vi "XY Graph Add Multiplots with Names v2.vi"(0 "XYGraph in":T3, 1 "Array of Scales (Default)":cluster{"X Scale":u32, "Y Scale":u32}[](array[cluster]), 2 "Plots Interpolation (Previous Plot's Style)":T2[](array[typedef]), 3 "Keep Existing Plots (T)":bool=TRUE, 5 "Array of Plots":cluster{"X Array":dbl[], "Y Array":dbl[]}[](array[cluster]), 7 "Plots Metadata":variant[](array[variant]), 9 "Array of Plot Names (\"Plot\")":string[](array[string]), 11 "error in (no error)":errorcluster, 12 "Make Visible (T)":bool=TRUE, 13 "Plot Colors (Default)":u32[](array[colorbox]), 14 "Point Style (Dot)":T1=enum."Dot") -> (4 "XY Graph Caption (or Label)":string, 6 "Total Number of Plots":i32, 8 "Number of Plots Added":i32, 10 "Added Plot Names":string[](array[string]), 15 "error out":errorcluster)   [LabVIEW 2021, in "XY Graph Add-Ons.lvlib"]
uses:
  XY Graph Add-Ons.lvlib
  XY Graph Refnum.ctl
  LabVIEW Plot Interpolation.ctl
  Plot Point Style.ctl
  XY Graph Get Plots Metadata.vi
  XY Graph Set Plots Metadata.vi
  Strings/Strings.lvlib
  Graphs.lvlib
  Error/Error.lvlib
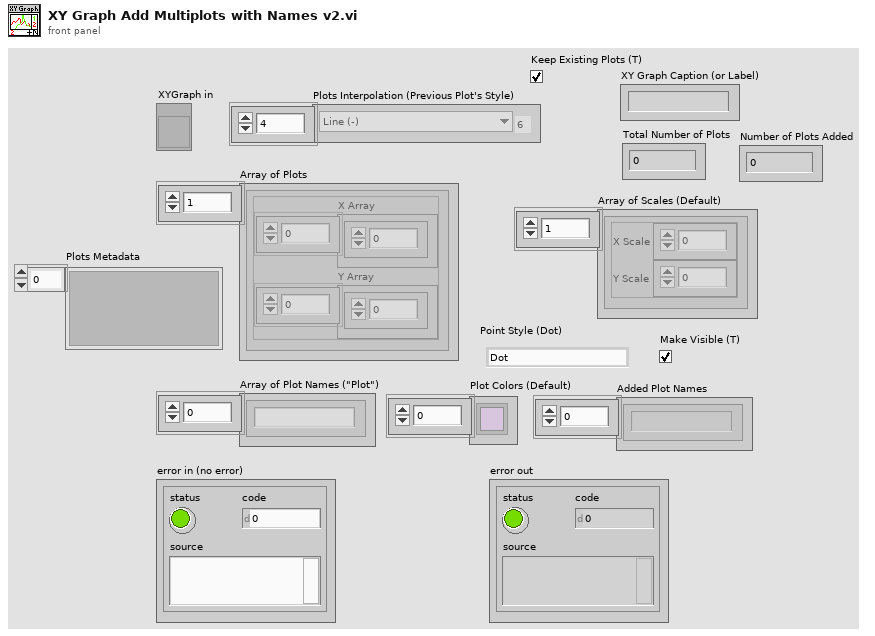
[diagram p1: front panel]
types:
  T1 = typedef "Graphs.lvlib/Plot Point Style.ctl" = enum16{"not defined", "None", "Empty Circle", "Filled Circle", "Thick Circle", "Dotted Circle", "Empty Square", "Filled Square", "Thick Square", "Dotted Square", "Small Filled Square", "Dot", "Cross", "Tiny Cross", "Large X", "Small x", "Diamond", "Small Empty Square"}
  T2 = typedef "Graphs.lvlib/LabVIEW Plot Interpolation.ctl" = enum16{"Point (.)", "Stepwise Right (--.)", "Line + Point (\\. /)", "Stepwise Left (.--)", "Stepwise Centered (-.-)", "Stepwise Vertical (|.|)", "Line (-)", "Use Previous Plot's Style"}
  T3 = typedef "XY Graph Add-Ons.lvlib/XY Graph Refnum.ctl" = refnum<vi>
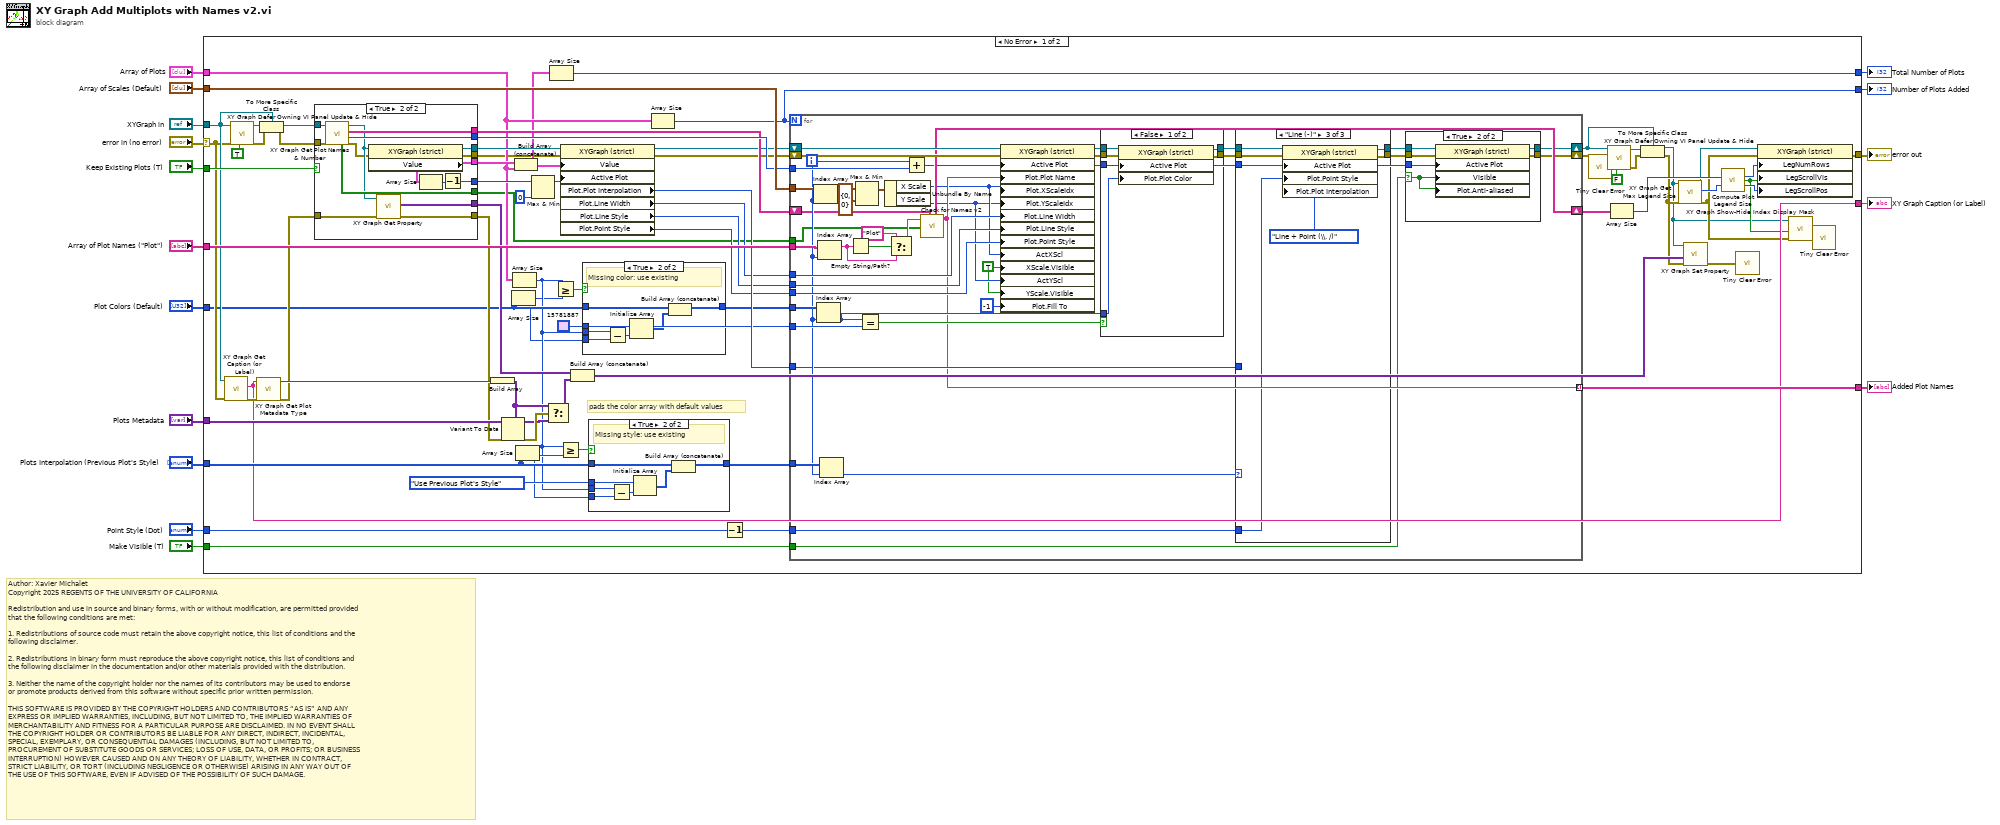
[diagram p0: block diagram]
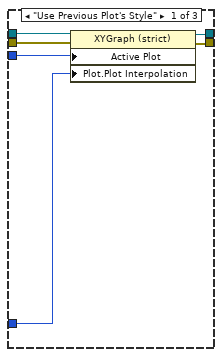
[diagram p4: hidden frame]
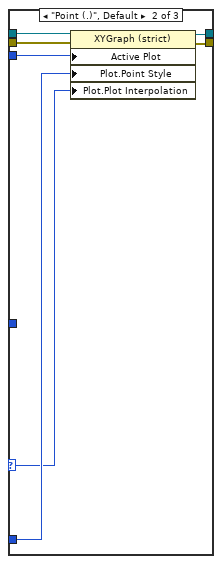
[diagram p5: hidden frame]
diagram:
  # "Author: Xavier Michalet\nCopyright 2025 REGENTS OF THE UNIVERSITY OF CALIFORNIA\n\nRedistribution and use in source and binary forms, with or without modification, are permitted provided\nthat the following conditions are met:\n\n1. Redistributions of source code must retain the above copyright notice, this list of conditions and the\nfollowing disclaimer.\n\n2. Redistributions in binary form must reproduce the above copyright notice, this list of conditions and\nthe following disclaimer in the documentation and/or other materials provided with the distribution.\n\n3. Neither the name of the copyright holder nor the names of its contributors may be used to endorse \nor promote products derived from this software without specific prior written permission.\n\nTHIS SOFTWARE IS PROVIDED BY THE COPYRIGHT HOLDERS AND CONTRIBUTORS “AS IS” AND ANY \nEXPRESS OR IMPLIED WARRANTIES, INCLUDING, BUT NOT LIMITED TO, THE IMPLIED WARRANTIES OF\nMERCHANTABILITY AND FITNESS FOR A PARTICULAR PURPOSE ARE DISCLAIMED. IN NO EVENT SHALL\nTHE COPYRIGHT HOLDER OR CONTRIBUTORS BE LIABLE FOR ANY DIRECT, INDIRECT, INCIDENTAL, \nSPECIAL, EXEMPLARY, OR CONSEQUENTIAL DAMAGES (INCLUDING, BUT NOT LIMITED TO, \nPROCUREMENT OF SUBSTITUTE GOODS OR SERVICES; LOSS OF USE, DATA, OR PROFITS; OR BUSINESS\nINTERRUPTION) HOWEVER CAUSED AND ON ANY THEORY OF LIABILITY, WHETHER IN CONTRACT, \nSTRICT LIABILITY, OR TORT (INCLUDING NEGLIGENCE OR OTHERWISE) ARISING IN ANY WAY OUT OF\nTHE USE OF THIS SOFTWARE, EVEN IF ADVISED OF THE POSSIBILITY OF SUCH DAMAGE."
  n1 = case shown="No Error" "error in (no error)" {
    selector: "error in (no error)" -> [w32 w204]
    tunnel: "XYGraph in" -> [w42 _]
    tunnel: "Array of Plot Names (\"Plot\")" -> [w89 _]
    tunnel: "Array of Scales (Default)" -> [w88 _]
    tunnel: [w79 _] -> w12
    tunnel: "Array of Plots" -> [w78 _]
    tunnel: "Plot Colors (Default)" -> [w22 _]
    tunnel: "Plots Interpolation (Previous Plot's Style)" -> [w77 _]
    tunnel: "Keep Existing Plots (T)" -> [w72 _]
    tunnel: [w71 w204] -> w7
    tunnel: [w69 _] -> w6
    tunnel: "Point Style (Dot)" -> [w68 _]
    tunnel: "Make Visible (T)" -> [w66 _]
    tunnel: [w64 _] -> w3
    tunnel: [w30 _] -> w2
    tunnel: "Plots Metadata" -> [w40 _]
    frame No Error {
      w20 = u32 15781887 ("Plot Color (Default)")
      # "pads the color array with default values"
      n2 = call "XY Graph Get Caption (or Label).vi"("error in (no error)"=w32, "XY Graph in"=w42) -> ("error out"=w31:errorcluster, "Caption (or Label) Text"=w30:string)  [unwired: 7 in, 1 out]
      n3 = call "XY Graph Defer Owning VI Panel Update & Hide.vi"("Defer Owning Panel Update"=TRUE, "error in (no error)"=w32, "XY Graph Refnum in"=w42) -> ("error out"=w55:errorcluster, "XY Graph Refnum out"=w58:refnum<vi>)  [unwired: 7 in]
      n4 = call "XY Graph Get Plot Metadata Type.vi"("Error In"=w31, "Graph Label"=w30) -> ("Error Out"=w35:errorcluster, "Plot Metadata Type"=w41:variant)  [unwired: 7 in, 1 out]
      n5 = To More Specific Class(target class=w42, reference=w58, error in=w55) -> (specific class reference=w56:T3, error out=w54:errorcluster)
      n6 = case shown="True" w72 {
        tunnel: [w180 w195] -> w90
        tunnel: w56 -> [w180 w194]
        tunnel: w54 -> [w179 w193]
        tunnel: [_ w192] -> w87
        tunnel: [_ w190] -> w86
        tunnel: [_ w189] -> w85
        tunnel: [_ w188] -> w84
        tunnel: [w179 w187] -> w65
        tunnel: [_ w186] -> w57
        tunnel: [_ w184] -> w45
        tunnel: w35 -> [w178 w182]
        tunnel: [w178 w181] -> w34
        frame False {
        }
        frame True {
          n7 = call "XY Graph Get Plot Names & Number.vi"("error in (no error)"=w193, "XYGraph in"=w194) -> ("error out"=w183:errorcluster, "# Plots"=w189:i32, "Plot Names"=w188:string[], "XYGraph out"=w185:T3, "Empty Plots?"=w186:bool[])  [unwired: 4 in, 1 out]
          n8 = property class="XYGraph (strict)"(reference=w185, error in=w183) -> (reference out=w195:T3, error out=w187:errorcluster, "Value"=w192:cluster{"X Array":dbl[], "Y Array":dbl[]}[])
          n9 = call-poly "XY Graph Get Property.vi"("Error In"=w182, "XYGraph Ref"=w185) -> ("Error Out"=w181:errorcluster, "Plot Metadata"=w184:variant[])  [unwired: 6 in, 2 out]
          n10 = Array Size(array=w192) -> (size(s)=w191:i32)
          n11 = Decrement(x=w191) -> (x-1=w190:i32)
        }
      }
      n12 = Build Array(w41) -> (w37:variant[])
      n13 = Variant To Data(error in=w34, type=w37, Variant=w40) -> (data=w38:variant[], error out=w39:errorcluster)
      n14 = Array Size(array=w22) -> (size(s)=w18:i32)
      n15 = Array Size(array=w78) -> (size(s)=w19:i32)
      n16 = Build Array (concatenate)(w87, w78) -> (w70:cluster{"X Array":dbl[], "Y Array":dbl[]}[])
      n17 = Array Size(array=w77) -> (size(s)=w24:i32)
      n18 = Max & Min(x=w86, y=0) -> (max(x,y)=w74:i32)  [unwired: 1 out]
      n19 = Select(t=w37, s=w39, f=w38) -> (s? t:f=w36:variant[])
      n20 = Array Size(array=w70) -> (size(s)=w69:i32)
      n21 = Greater Or Equal?(x=w19, y=w18) -> (x >= y?=w23:bool)
      n22 = Greater Or Equal?(x=w19, y=w24) -> (x >= y?=w25:bool)
      n23 = property class="XYGraph (strict)"(reference=w90, error in=w65, "Value"=w70, "Active Plot"=w74) -> (reference out=w63:T3, error out=w62:errorcluster, "Plot.Plot Interpolation"=w83:u8, "Plot.Line Width"=w82:u8, "Plot.Line Style"=w81:u8, "Plot.Point Style"=w80:u8)
      n24 = Build Array (concatenate)(w45, w36) -> (w44:variant[])
      n25 = case shown="True" w23 {
        tunnel: w22 -> [w92 w99]
        tunnel: [w92 w98] -> w21
        tunnel: w20 -> [_ w96]
        tunnel: w19 -> [_ w95]
        tunnel: w18 -> [_ w94]
        frame False {
        }
        frame True {
          # "Missing color: use existing"
          n26 = Subtract(x=w95, y=w94) -> (x-y=w97:i32)
          n27 = Initialize Array(w96, w97) -> (w93:u32[])
          n28 = Build Array (concatenate)(w99, w93) -> (w98:u32[])
        }
      }
      n29 = case shown="True" w25 {
        tunnel: w77 -> [w196 w203]
        tunnel: [w196 w202] -> w76
        tunnel: LabVIEW_Plot_Interpolation."Use Previous Plot's Style" ("Plot Interpolation") -> [_ w200]
        tunnel: w19 -> [_ w199]
        tunnel: w24 -> [_ w198]
        frame False {
        }
        frame True {
          # "Missing style: use existing"
          n30 = Subtract(x=w199, y=w198) -> (x-y=w197:i32)
          n31 = Initialize Array(w200, w197) -> (w201:T2[])
          n32 = Build Array (concatenate)(w203, w201) -> (w202:T2[])
        }
      }
      n33 = Array Size(array=w78) -> (size(s)=w64:i32)
      n34 = Decrement(x=w68) -> (x-1=w67:T1)
      n35 = for {
        N: w64 -> [_]
        tunnel: w89 -> [w138]
        shift-right: [w109] -> w61
        shift-left: w62 -> [w140]
        shift-right: [w112] -> w47
        shift-left: w63 -> [w141]
        tunnel: w85 -> [w139]
        shift-right: [w115] -> w91
        shift-left: w84 -> [w116]
        tunnel: w88 -> [w137]
        tunnel: w83 -> [w118]
        tunnel: w82 -> [w132]
        tunnel: w81 -> [w131]
        tunnel: w80 -> [w130]
        tunnel: [w113] -> w79 mode=indexing
        tunnel: w21 -> [w129]
        tunnel: w20 -> [w128]
        tunnel: w76 -> [w120]
        tunnel: w67 -> [w117]
        tunnel: w66 -> [w111]
        tunnel: w57 -> [w105]
        i -> [w119]
        w102 = TRUE ("X Scale.Visible")
        n36 = Index Array(array=w137, index=w119) -> (element=w136:cluster{"X Scale":u32, "Y Scale":u32})
        n37 = Index Array(array=w129, index=w119) -> (element=w124:u32)
        n38 = Index Array(array=w138, index=w119) -> (element=w134:string)
        n39 = Index Array(array=w120, index=w119) -> (element=w100:T2)
        n40 = Empty String/Path?(string/path=w134) -> (empty?=w135:bool)
        n41 = Max & Min(x=w136, y=cluster{"X Scale":u32, "Y Scale":u32} {"X Scale"=0, "Y Scale"=0}) -> (max(x,y)=w107:cluster{"X Scale":u32, "Y Scale":u32})  [unwired: 1 out]
        n42 = Equal?(x=w124, y=w128) -> (x = y?=w127:bool)
        n43 = Unbundle By Name(w107) -> ("X Scale"=w104:u32, "Y Scale"=w103:u32)
        n44 = Select(t="Plot", s=w135, f=w134) -> (s? t:f=w114:string)
        n45 = Add(x=w119, y=w139) -> (x+y=w108:i32)
        n46 = call "Check for Names v2.vi"("New Name"=w114, "Name List"=w116, "Empty Plots?"=w105) -> ("New Name List"=w115:string[], "New Name"=w113:string)  [unwired: 3 in, 2 out]
        n47 = property class="XYGraph (strict)"(reference=w141, error in=w140, "Active Plot"=w108, "Plot.Plot Name"=w113, "Plot.XScaleIdx"=w104, "Plot.YScaleIdx"=w103, "Plot.Line Width"=w132, "Plot.Line Style"=w131, "Plot.Point Style"=w130, "ActXScl"=w104, "XScale.Visible"=w102, "ActYScl"=w103, "YScale.Visible"=w102, "Plot.Fill To"=i16 -1) -> (reference out=w126:T3, error out=w125:errorcluster)
        n48 = case shown="False" w127 {
          tunnel: w126 -> [w175 w177]
          tunnel: [w174 w177] -> w123
          tunnel: w125 -> [w173 w176]
          tunnel: [w172 w176] -> w122
          tunnel: w124 -> [w171 _]
          tunnel: w108 -> [w170 _]
          frame False {
            n49 = property class="XYGraph (strict)"(reference=w175, error in=w173, "Active Plot"=w170, "Plot.Plot Color"=w171) -> (reference out=w174:T3, error out=w172:errorcluster)
          }
          frame True {
          }
        }
        n50 = case shown="\"Line (-)\"" w100 {
          selector: w100 -> [_ w156 _]
          tunnel: w123 -> [w155 w162 w169]
          tunnel: [w154 w161 w168] -> w121
          tunnel: w122 -> [w153 w160 w167]
          tunnel: [w152 w159 w166] -> w110
          tunnel: w108 -> [w151 w158 w165]
          tunnel: w118 -> [w150 _ _]
          tunnel: w117 -> [_ w157 w164]
          frame "Use Previous Plot's Style" {
            n51 = property class="XYGraph (strict)"(reference=w155, error in=w153, "Active Plot"=w151, "Plot.Plot Interpolation"=w150) -> (reference out=w154:T3, error out=w152:errorcluster)
          }
          frame "Point (.)", Default {
            n52 = property class="XYGraph (strict)"(reference=w162, error in=w160, "Active Plot"=w158, "Plot.Point Style"=w157, "Plot.Plot Interpolation"=w156) -> (reference out=w161:T3, error out=w159:errorcluster)
          }
          frame "Line (-)" {
            n53 = property class="XYGraph (strict)"(reference=w169, error in=w167, "Active Plot"=w165, "Plot.Point Style"=w164, "Plot.Plot Interpolation"=LabVIEW_Plot_Interpolation."Line + Point (\\. /)" ("Plot Interpolation")) -> (reference out=w168:T3, error out=w166:errorcluster)
          }
        }
        n54 = case shown="True" w111 {
          selector: w111 -> [_ w144]
          tunnel: w121 -> [w143 w149]
          tunnel: [w143 w148] -> w112
          tunnel: w110 -> [w142 w147]
          tunnel: [w142 w146] -> w109
          tunnel: w108 -> [_ w145]
          frame False {
          }
          frame True {
            n55 = property class="XYGraph (strict)"(reference=w149, error in=w147, "Active Plot"=w145, "Visible"=w144, "Plot.Anti-aliased"=w144) -> (reference out=w148:T3, error out=w146:errorcluster)
          }
        }
      }
      n56 = call "Tiny Clear Error.vi"("Error In"=w61) -> ("no Error Out"=w17:errorcluster)  [unwired: 8 in]
      n57 = call "XY Graph Defer Owning VI Panel Update & Hide.vi"("Defer Owning Panel Update"=FALSE, "error in (no error)"=w17, "XY Graph Refnum in"=w47) -> ("error out"=w49:errorcluster, "XY Graph Refnum out"=w48:refnum<vi>)  [unwired: 7 in]
      n58 = Array Size(array=w91) -> (size(s)=w52:i32)
      n59 = To More Specific Class(target class=w47, reference=w48, error in=w49) -> (specific class reference=w26:T3, error out=w43:errorcluster)
      n60 = call "XY Graph Get Max Legend Size.vi"("Error In"=w43, "XYGraph Refnum"=w26) -> ("Error Out"=w28:errorcluster, "Max Legend Size"=w53:i32, "XYGraph Refnum"=w46:T3)  [unwired: 6 in, 1 out]
      n61 = call-poly "XY Graph Set Property.vi"("error in (no error)"=w43, "Plots Metadata"=w44, "XY Graph Refnum"=w26) -> ("error out"=w33:errorcluster)  [unwired: 7 in, 1 out]
      n62 = call "Compute Plot Legend Size.vi"("# Plots"=w52, "Max Legend Size"=w53) -> ("LegNumRows"=w51:u32, "LegScrollVis"=w27:bool, "LegScrollPos"=w50:u32)  [unwired: 11 in]
      n63 = call "Tiny Clear Error.vi"("Error In"=w33) -> ()  [unwired: 8 in, 1 out]
      n64 = property class="XYGraph (strict)"(reference=w46, error in=w28, "LegNumRows"=w51, "LegScrollVis"=w27, "LegScrollPos"=w50) -> (error out=w71:errorcluster)  [unwired: 1 out]
      n65 = call "XY Graph Show-Hide Index Display Mask.vi"("error in (no error)"=w28, "Show(T)/Hide(F)"=w27, "XYGraph Ref"=w26) -> ("error out"=w29:errorcluster)  [unwired: 7 in, 1 out]
      n66 = call "Tiny Clear Error.vi"("Error In"=w29) -> ()  [unwired: 8 in, 1 out]
    }
    frame Error {
    }
  }
  "error out" <- w7
  "Added Plot Names" <- w12
  "Total Number of Plots" <- w6
  "Number of Plots Added" <- w3
  "XY Graph Caption (or Label)" <- w2
